vi "Calculate Mask Test Gate.vi"(6 "Stop":dbl, 7 "Start":dbl, 8 "error in":errorcluster, 9 "Gate Type":i32(ring) items=["Time", "Points", "Frequency", "Cursors"], 10 "Calculation Channel":i32(ring) items=["Calc Channel 1", "Calc Channel 2", "Calc Channel 3", "Calc Channel 4"], 11 "Instrument Handle In":i32) -> (0 "error out":errorcluster, 3 "Instrument Handle Out":i32)   [LabVIEW 8.6, in "ZTScopeM.lvlib"]
doc: "Configure the gating for masks tests on the selected channel."
uses:
  ZTScopeM.lvlib
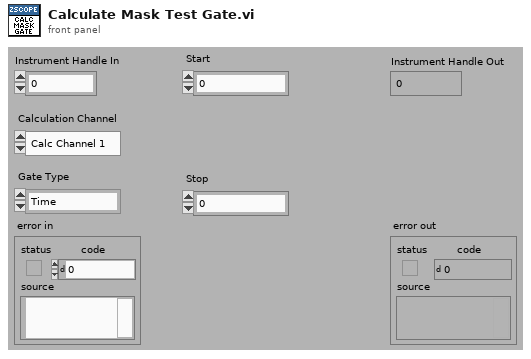
[diagram p1: front panel]
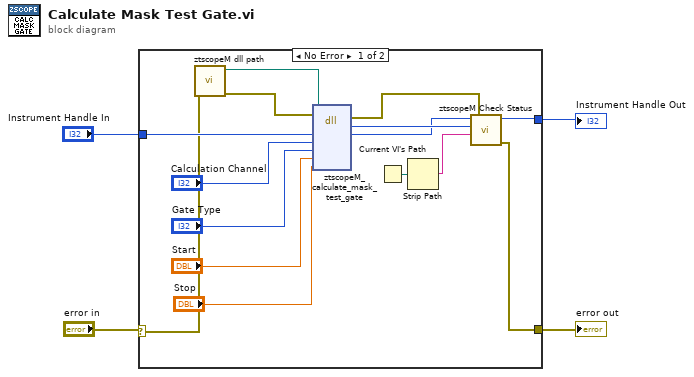
[diagram p0: block diagram]
diagram:
  n1 = case shown="No Error" "error in" {
    selector: "error in" -> [w8 w21]
    tunnel: [w10 w21] -> w1
    tunnel: "Instrument Handle In" -> [w19 w20]
    tunnel: [w11 w20] -> w3
    frame #0 {
      n2 = call "ztscopeM dll path.vi"("error in (no error)"=w8) -> ("error out"=w6:errorcluster, "<instrument>.dll path"=w7:path)  [unwired: 9 in]
      n3 = dll-call lib="C:/Program Files (x86)/National Instruments/LabVIEW 2013/instr.lib/ztscopem/ztscopeM.dll" fn="ztscopeM_calculate_mask_test_gate"(path in=w7, error in=w6, "instrumentHandle"=w19, "calculationChannel"="Calculation Channel", "gate type"="Gate Type", "start"="Start", "stop"="Stop") -> (error out=w5:errorcluster, w13:i32, "instrumentHandle"=w12:i32)  [unwired: 5 in, 1 out]
      n4 = Current VI's Path() -> (path=w15:path)
      n5 = Strip Path(path=w15) -> (name=w14:string)  [unwired: 1 out]
      n6 = call "ztscopeM Check Status.vi"("error in"=w5, "name of VI"=w14, "status (return code)"=w13, "instrument handle in"=w12) -> ("error out"=w10:errorcluster, "instrument handle out"=w11:i32)  [unwired: 2 in]
    }
    frame #1 {
    }
  }
  "Instrument Handle Out" <- w3
  "error out" <- w1
